vi "config2.vi"() -> (0 "thin Film 1":dbl=1.3668, 1 "DSSC1_WP":dbl, 2 "DSSC2_WP":dbl, 3 "DSSC3_WP":dbl, 4 "thin Film 2":dbl=1.3668, 5 "Poly Si 2":dbl=1.3668, 6 "THINFILM2_WP":dbl, 7 "THINFILM1_WP":dbl, 8 "POLYSI2_WP":dbl, 9 "POLYSI1_WP":dbl, 13 "Poly Si 1":dbl=1.3668, 14 "DSSC 2":dbl=0.01296, 15 "DSSC 1":dbl=0.375, 18 "path":path, 19 "DSSC3":dbl=1.0)   [LabVIEW 2012]
panel:
  in  "POLYSI2_WP":dbl=50.0
  in  "POLYSI1_WP":dbl=50.0
  in  "THINFILM2_WP":dbl=30.0
  in  "THINFILM1_WP":dbl=30.0
  in  "DSSC3_WP":dbl=2.0
  in  "DSSC2_WP":dbl=0.123
  in  "DSSC1_WP":dbl=0.04
  in  "Poly Si 2":dbl=0.357
  in  "Poly Si 1":dbl=0.357
  in  "Thin film 2":dbl=0.6
  in  "DSSC 3":dbl=0.366
  in  "Thin film 1":dbl=0.6
  in  "DSSC 2":dbl=0.288
  in  "DSSC 1":dbl=0.3
  in  "Start":bool
  in  "Save in":path=path "C:/Measurements"
  # "Area of the cell(m2)"
  # "Wp(Watt)"
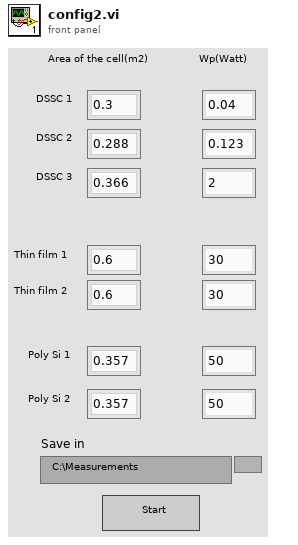
[diagram p1: front panel]
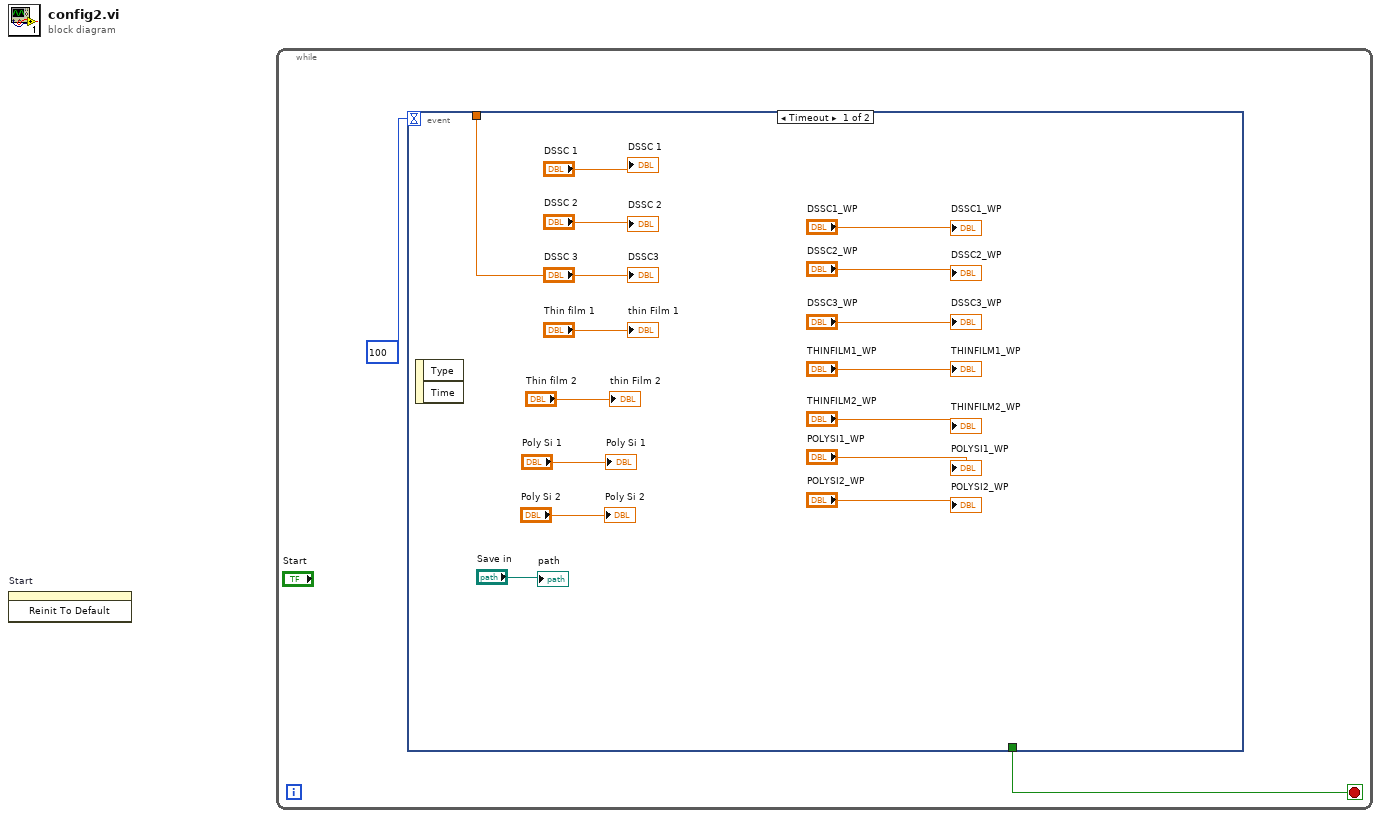
[diagram p0: block diagram]
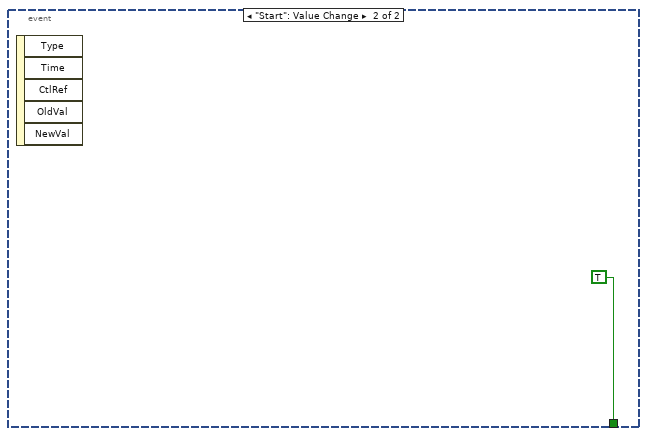
[diagram p2: hidden frame]
diagram:
  n1 = invoke on="Start" class="Bool" method="Reinit To Default"() -> ()  [unwired: 3 in, 3 out]
  n2 = while {
    stop <- w2 stop-if-true
    n3 = event shown="[0] Timeout" {
      selector: _ -> [_ _]
      dyn-events: _ -> [_ _]
      timeout: 100 -> [_ _]
      tunnel: [_ TRUE] -> w2
      tunnel: ["DSSC 3" _] -> _
      event Timeout {
        n4 = event-data() -> ()  [unwired: 1 in, 2 out]
        "path" <- "Save in"
        "DSSC 1" <- "DSSC 1"
        "DSSC 2" <- "DSSC 2"
        "thin Film 1" <- "Thin film 1"
        "DSSC3" <- "DSSC 3"
        "thin Film 2" <- "Thin film 2"
        "Poly Si 1" <- "Poly Si 1"
        "Poly Si 2" <- "Poly Si 2"
        "DSSC1_WP" <- "DSSC1_WP"
        "DSSC2_WP" <- "DSSC2_WP"
        "DSSC3_WP" <- "DSSC3_WP"
        "THINFILM1_WP" <- "THINFILM1_WP"
        "THINFILM2_WP" <- "THINFILM2_WP"
        "POLYSI1_WP" <- "POLYSI1_WP"
        "POLYSI2_WP" <- "POLYSI2_WP"
      }
      event "Start": Value Change {
        n5 = event-data() -> ()  [unwired: 1 in, 5 out]
      }
    }
  }
